vi "Initialize RT.vi"(8 "error in":errorcluster) -> (0 "error out":errorcluster, 1 "Acceleration RT FIFO":T1, 3 "rt fifo":refnum<k33>)   [LabVIEW 2017]
doc: "Initialize shared variables and RT FIFOs and turn on RT LED."
uses:
  controls/Acceleration RT FIFO Reference.ctl
  <vilib>/vision/Image Controls.llb/IMAQ Image.ctl
  Globals/Global - Configuration Options.vi
  <vilib>/NI_Real-Time Target Support.lvlib
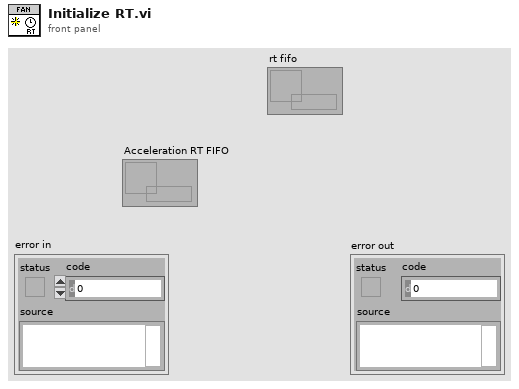
[diagram p1: front panel]
types:
  T1 = typedef "Acceleration RT FIFO Reference.ctl" = refnum<k33>
  T2 = typedef "IMAQ Image.ctl" = refnum<image>
  T3 = cluster{"read mode":enum16{"polling", "blocking"}, "write mode":enum16{"polling", "blocking"}}
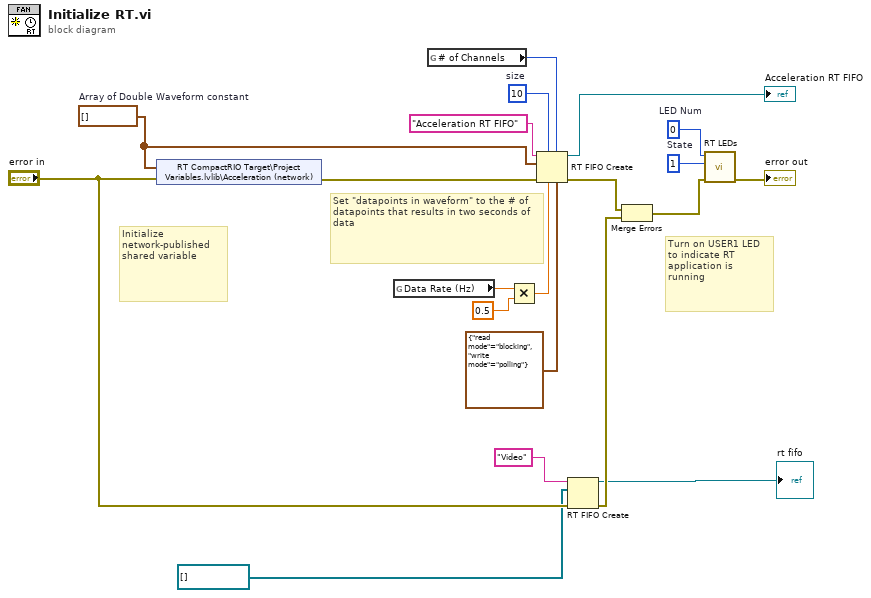
[diagram p0: block diagram]
diagram:
  w13 = waveform(dbl)[] []  # Array of Double Waveform constant
  w17 = u32 10  # size
  w18 = 1  # State
  w19 = 0  # LED Num
  # "Set \"datapoints in waveform\" to the # of datapoints that results in two seconds of data"
  # "Initialize network-published shared variable"
  # "Turn on USER1 LED to indicate RT application is running"
  n1 = shared-variable "RT CompactRIO Target\\Project Variables.lvlib\\Acceleration (network)"(w13, error in="error in") -> (error out=w15:errorcluster)
  n2 = global read "Global - Configuration Options.vi" "Data Rate (Hz)"() -> (w10:dbl)
  n3 = global read "Global - Configuration Options.vi" "# of Channels"() -> (w11:u32)
  n4 = Multiply(x=w10, y=0.5) -> (x*y=w8:dbl)
  n5 = RT FIFO Create(0:"Acceleration RT FIFO" ("name (unnamed)"), 1:w13, 3:w15, 4:w17, 5:w8, 6:w11, 7:T3 {"read mode"=enum."blocking", "write mode"=enum."polling"} ("r/w modes (polling,polling)")) -> (8:→"Acceleration RT FIFO":refnum<k33>, 11:w6:errorcluster)  [unwired: 1 in, 1 out]
  n6 = RT FIFO Create(0:"Video" ("name (unnamed)"), 1:T2[] [], 3:"error in") -> (8:→"rt fifo":refnum<k33>, 11:w5:errorcluster)  [unwired: 5 in, 1 out]
  n7 = Merge Errors(w6, w5) -> (w4:errorcluster)
  n8 = call <vilib>:"RT LEDs.vi"("error in (no error)"=w4, "State"=w18, "LED Num"=w19) -> ("error out"=→"error out":errorcluster)  [unwired: 3 in, 1 out]
